vi "motor monitoring.vi"(8 "error in":errorcluster, 9 "record":string="A", 10 "Value":string="A", 11 "IOC":string) -> (0 "error out":errorcluster, 3 "Moved":bool)   [LabVIEW 2022 SP3]
uses:
  pectus/global/global path.vi
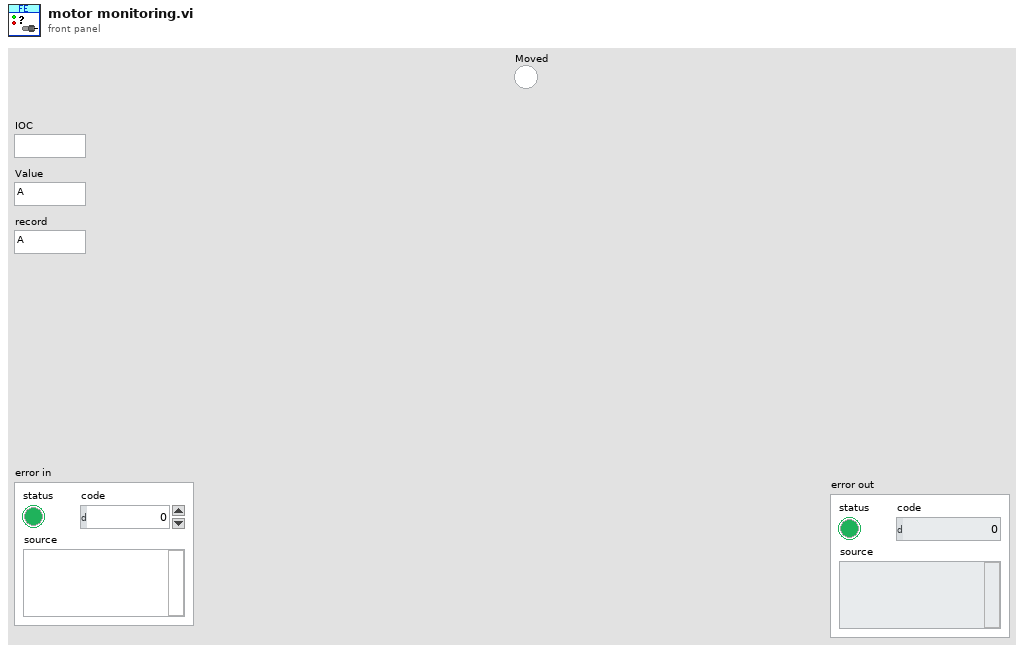
[diagram p1: front panel]
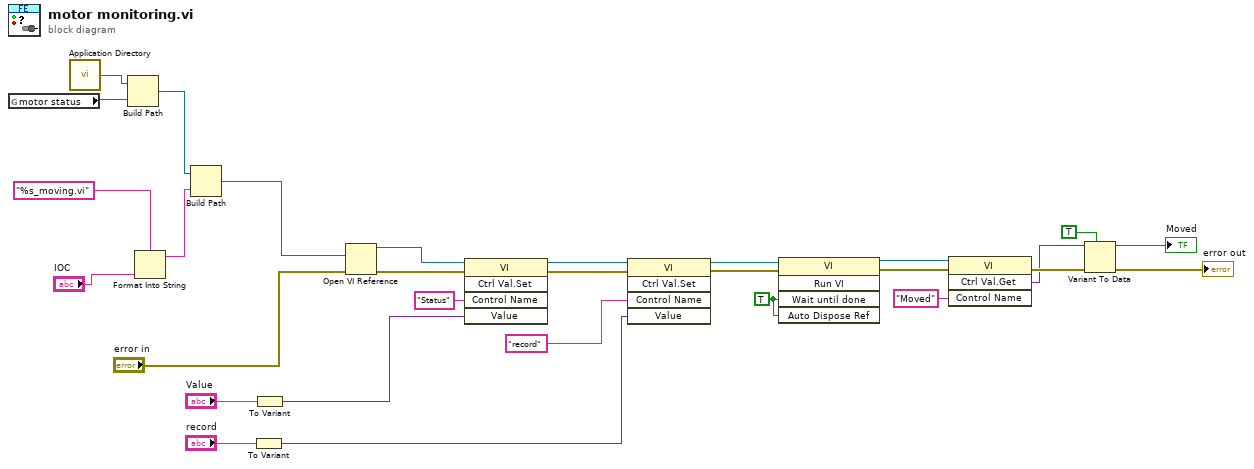
[diagram p0: block diagram]
diagram:
  w22 = TRUE ("Wait Until Done")
  n1 = global read "global path.vi" "motor status"() -> (w13:path)
  n2 = call <vilib>:"Application Directory.vi"() -> ("Application Directory"=w12:path)
  n3 = Build Path(base path=w12, name or relative path=w13) -> (appended path=w11:path)
  n4 = Format Into String(format string="%s_moving.vi", "IOC") -> (resulting string=w8:string)  [unwired: 2 in, 1 out]
  n5 = Build Path(base path=w11, name or relative path=w8) -> (appended path=w29:path)
  n6 = To Variant(anything="record") -> (Variant=w1:variant)
  n7 = To Variant(anything="Value") -> (Variant=w23:variant)
  n8 = Open VI Reference(vi path=w29, error in (no error)="error in") -> (vi reference=w27:refnum<vi>, error out=w26:errorcluster)  [unwired: 4 in]
  n9 = invoke class="VI" method="Ctrl Val.Set"(reference=w27, error in=w26, "Control Name"="Status", "Value"=w23) -> (reference out=w7:refnum<vi>, error out=w6:errorcluster)  [unwired: 1 in, 3 out]
  n10 = invoke class="VI" method="Ctrl Val.Set"(reference=w7, error in=w6, "Control Name"="record", "Value"=w1) -> (reference out=w5:refnum<vi>, error out=w4:errorcluster)  [unwired: 1 in, 3 out]
  n11 = invoke class="VI" method="Run VI"(reference=w5, error in=w4, "Wait until done"=w22, "Auto Dispose Ref"=w22) -> (reference out=w21:refnum<vi>, error out=w20:errorcluster)  [unwired: 1 in, 3 out]
  n12 = invoke class="VI" method="Ctrl Val.Get"(reference=w21, error in=w20, "Control Name"="Moved") -> (error out=w18:errorcluster, "Get Control Value Variant"=w17:variant)  [unwired: 1 in, 2 out]
  n13 = Variant To Data(error in=w18, type=TRUE, Variant=w17) -> (data=→"Moved":bool, error out=→"error out":errorcluster)
